vi "NXTCam-DM.vi"(0 "Input of NXTCam":T2={"Tracking Mode"=0, "Object Number to Track"=0, "Address"=2} {"Address" format="%x"; "Object Number to Track" format="%x"; "Tracking Mode" items=["Disable Tracking", "Get First Object", "Get n th Object", "Enable Tracking", "Sort Objects  by size", "Sort Objects  by Colors", "Illumination on ", "Illumination Off", "Write Colormap", "Read Colormap", "Line tracking mode", "Object Tracking mode"]}, 2 "NXT":T3={"Hardware"="NXT", "Flattened String"=""}, 3 "Input Port":T4 items=["Port 1", "Port 2", "Port 3", "Port 4"]) -> (1 "Output of NXTCam":T1, 4 "NXT dup":T3={"Hardware"="NXT", "Flattened String"=""} caption="NXT")   [LabVIEW 2011]
uses:
  <vilib>/NXT/Subs/LVHSConnector.ctl
  <vilib>/NXT/Block Support/NXT_InputPort.ctl
  <vilib>/NXT/Block Support/HWPage.SensorType.ctl
  <vilib>/NXT/Block Support/HWPage.SensorMode.ctl
panel:
  in  "Colormap Array":string="\u0000\u0000\u0000\u0000\u0000\u0000\u0000\u0000\u0000\u0000\u0000\u0000€€€€\u0000\u0000\u0000\u0000\u0000\u0000\u0000\u0000\u0000\u0000\u0000\u0000€€€€\u0000\u0000\u0000\u0000\u0000\u0000\u0000\u0000\u0000\u0000\u0000\u0000€€€€"
  in  "camera setting array":string="\u0000\u0000\u0000\u0000\u0000\u0000\u0000\u0000\u0000\u0000\u0000\u0000€€€€\u0000\u0000\u0000\u0000\u0000\u0000\u0000\u0000\u0000\u0000\u0000\u0000€€€€\u0000\u0000\u0000\u0000\u0000\u0000\u0000\u0000\u0000\u0000\u0000\u0000€€€€"
  out "Status (boolean)":bool
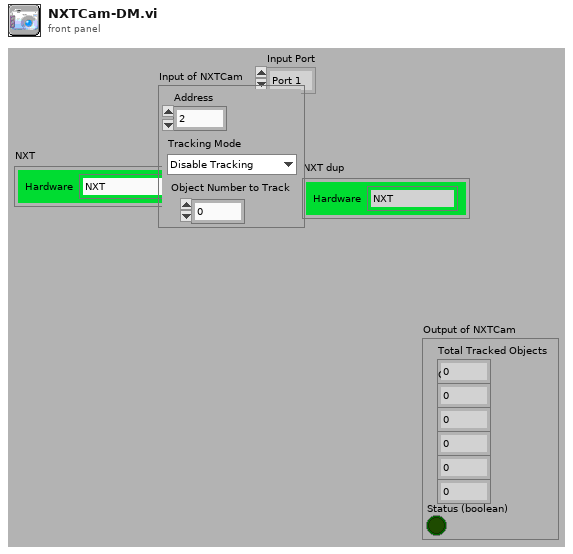
[diagram p1: front panel]
types:
  T1 = cluster{"Total Tracked Objects":u8, "Color":u8, "X Upper Left":u8, "Y Upper Left":u8, "X Lower Right":u8, "Y Lower Right":u8, "Status (boolean)":bool}
  T2 = cluster{"Tracking Mode":u8, "Object Number to Track":u8, "Address":u8}
  T3 = typedef "LVHSConnector.ctl" = cluster{"Hardware":string, "Flattened String":string}
  T4 = typedef "NXT_InputPort.ctl" = u8
  T5 = typedef "HWPage.SensorType.ctl" = u8
  T6 = typedef "HWPage.SensorMode.ctl" = u8
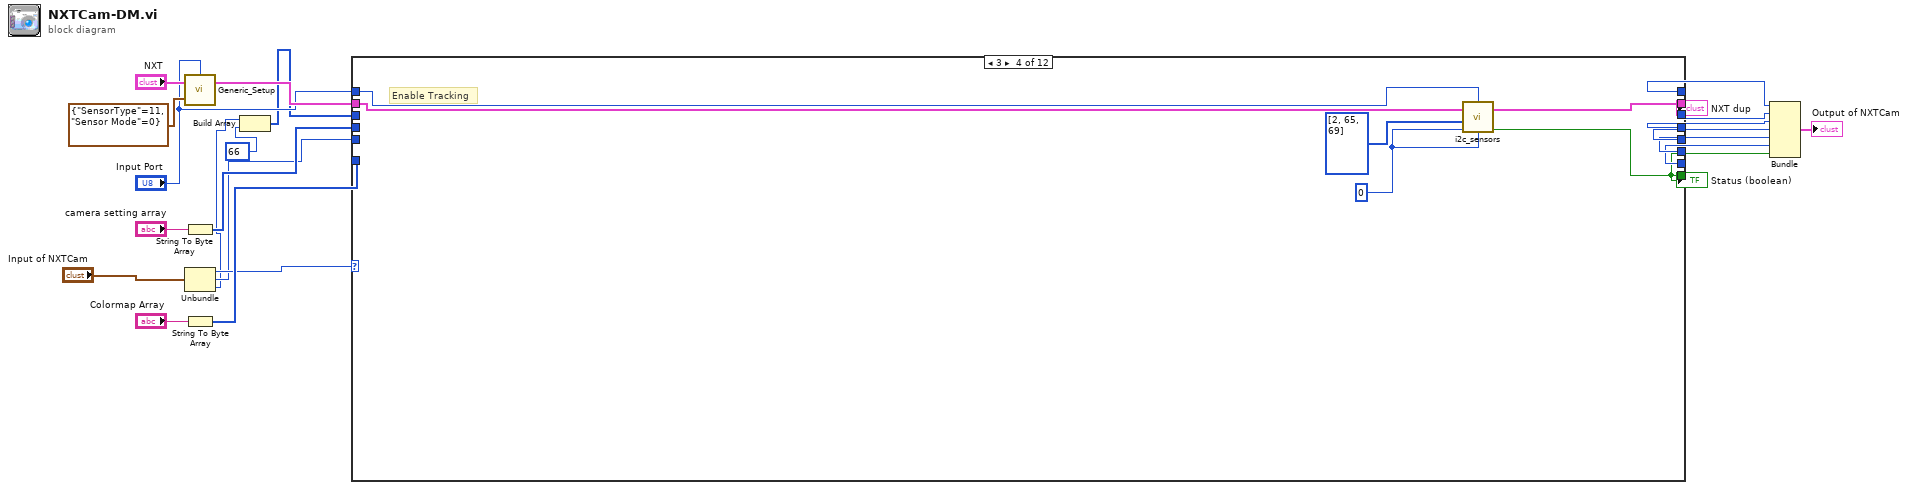
[diagram p0: block diagram]
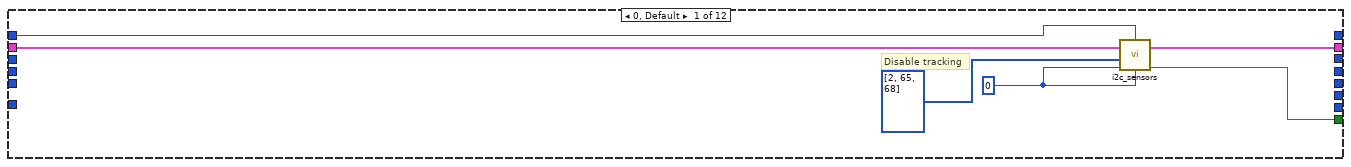
[diagram p2: hidden frame]
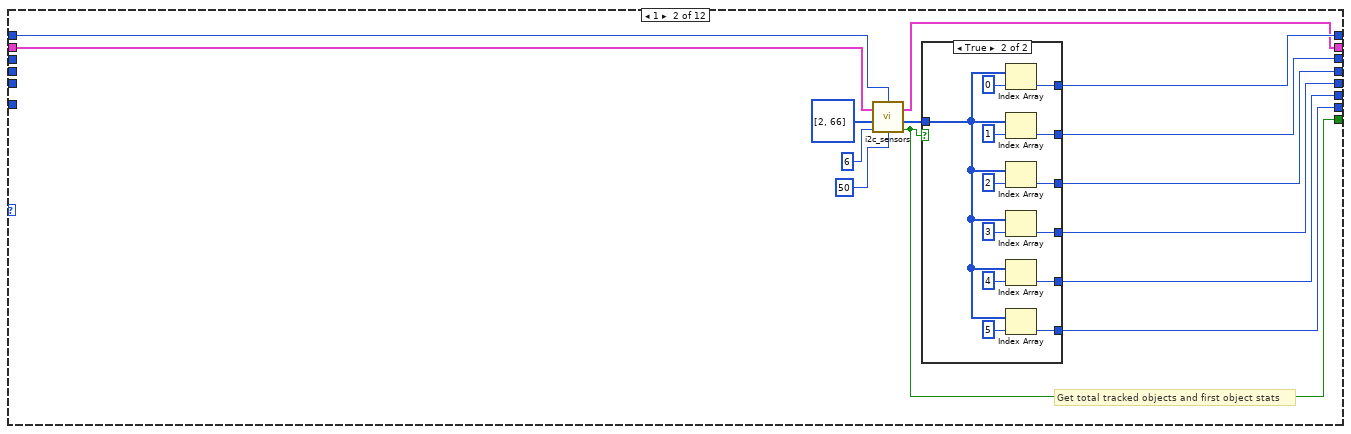
[diagram p3: hidden frame]
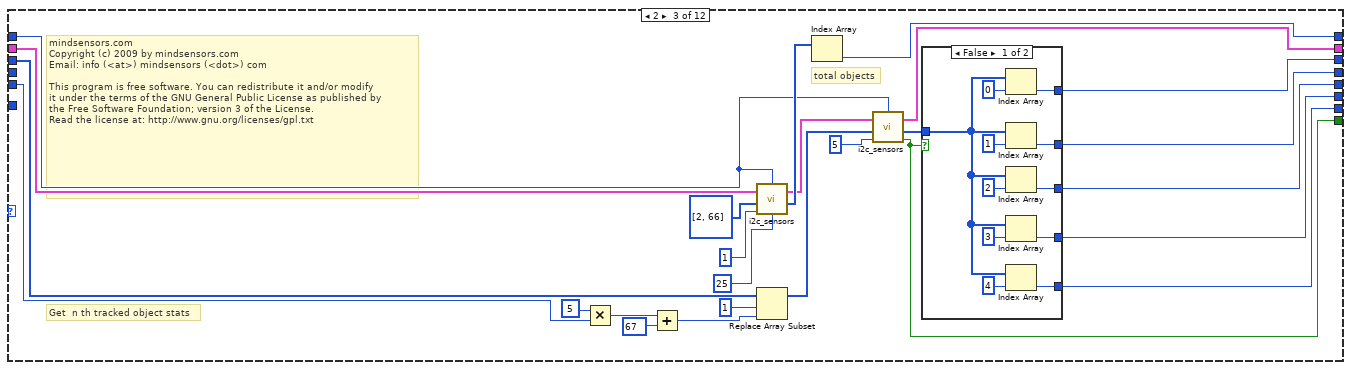
[diagram p5: hidden frame]
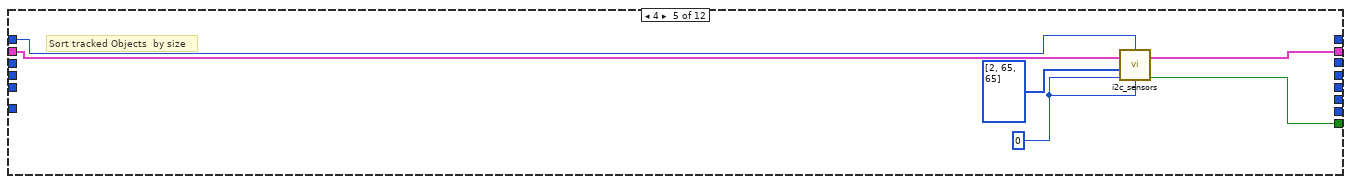
[diagram p7: hidden frame]
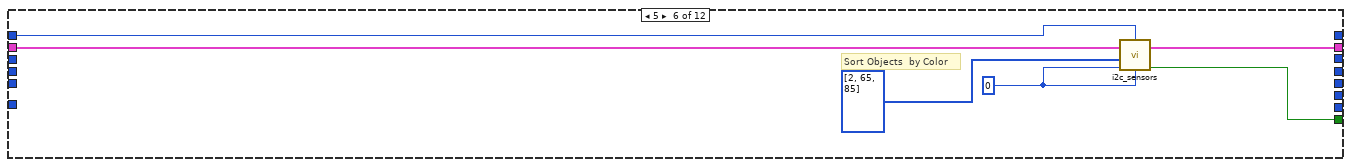
[diagram p8: hidden frame]
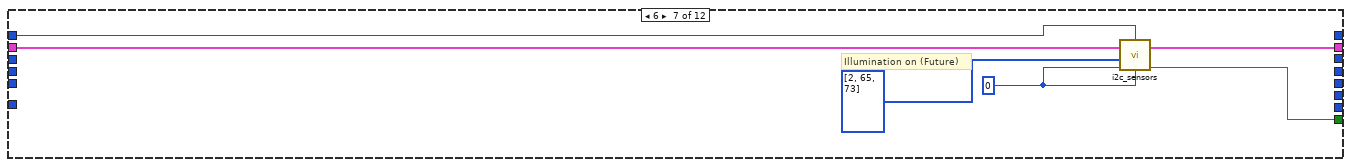
[diagram p9: hidden frame]
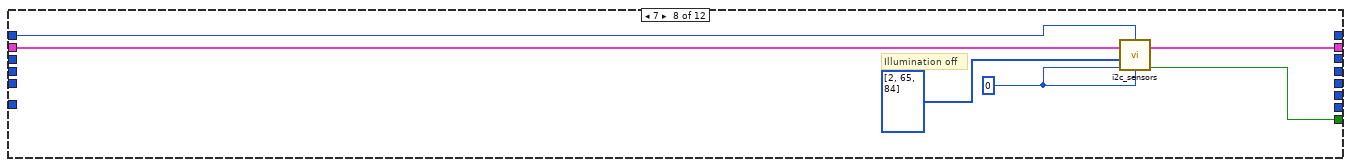
[diagram p10: hidden frame]
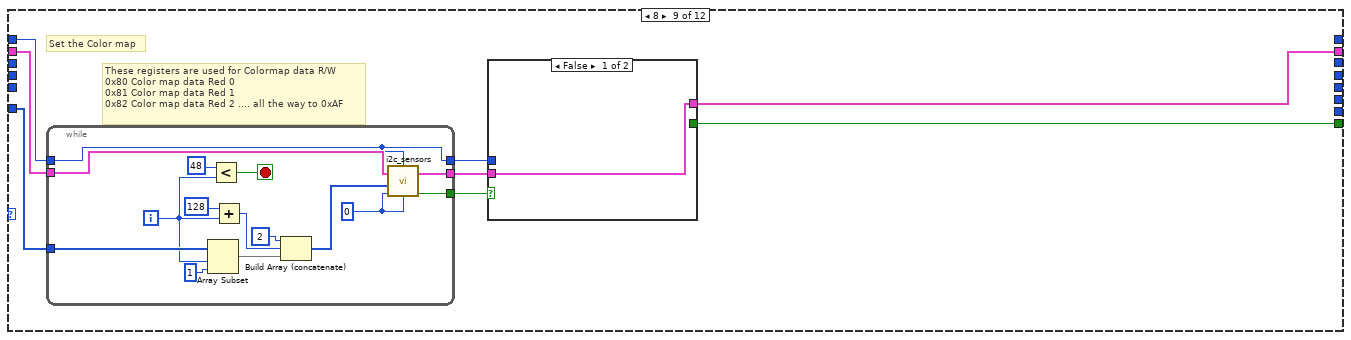
[diagram p11: hidden frame]
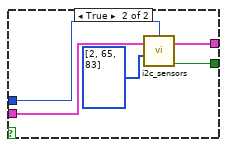
[diagram p12: hidden frame]
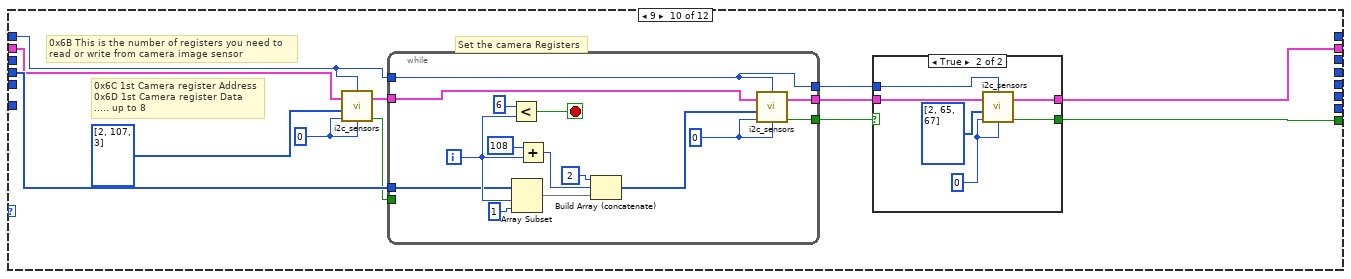
[diagram p13: hidden frame]
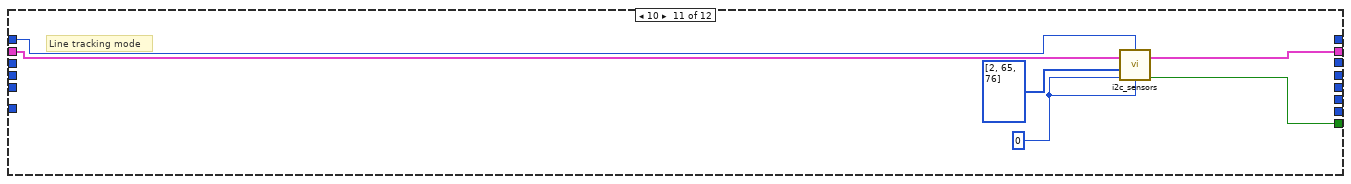
[diagram p15: hidden frame]
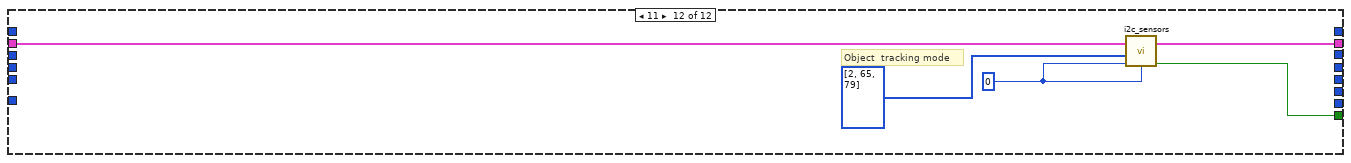
[diagram p16: hidden frame]
diagram:
  n1 = call <vilib>:"Generic_Setup.vi"("Sensor Setup"=cluster{"SensorType":T5, "Sensor Mode":T6} {"SensorType"=11, "Sensor Mode"=0}, "NXT"="NXT", "Port"="Input Port") -> ("NXT"=w15:T3)  [unwired: 1 out]
  n2 = String To Byte Array(string="camera setting array") -> (unsigned byte array=w17:u8[])
  n3 = Unbundle("Input of NXTCam") -> ("Tracking Mode"=w9:u8, "Object Number to Track"=w6:u8, "Address"=w3:u8)
  n4 = String To Byte Array(string="Colormap Array") -> (unsigned byte array=w16:u8[])
  n5 = Build Array(w3, 66 ("Slope")) -> (w1:i32[])
  n6 = case shown="3" w9 {
    tunnel: [w26 w31 w60 w94 w100 w106 w112 w118 w129 w161 w191 w193] -> w5
    tunnel: [_ w43 w70 _ _ _ _ _ _ _ _ _] -> w21
    tunnel: [_ w42 w75 _ _ _ _ _ _ _ _ _] -> w20
    tunnel: [_ w41 w74 _ _ _ _ _ _ _ _ _] -> w19
    tunnel: [_ w40 w73 _ _ _ _ _ _ _ _ _] -> w18
    tunnel: [_ w39 w72 _ _ _ _ _ _ _ _ _] -> w14
    tunnel: [_ w38 w71 _ _ _ _ _ _ _ _ _] -> w13
    tunnel: w1 -> [_ _ w76 _ _ _ _ _ _ _ _ _]
    tunnel: w16 -> [_ _ _ _ _ _ _ _ w130 _ _ _]
    tunnel: w17 -> [_ _ _ _ _ _ _ _ _ w163 _ _]
    tunnel: "Input Port" -> [w27 w33 w59 w97 w102 w107 w113 w120 w127 w157 w189 _]
    tunnel: w15 -> [w29 w36 w69 w98 w103 w110 w114 w122 w126 w159 w192 w196]
    tunnel: [w24 w35 w62 w95 w101 w109 w115 w121 w124 w152 w190 w197] -> w12
    tunnel: w6 -> [_ _ w57 _ _ _ _ _ _ _ _ _]
    frame 0, Default {
      w25 = u8 0 ("Return Length")
      # "Disable tracking"
      n7 = call <vilib>:"i2c_sensors.vi"("Return Length"=w25, "Bytes to Write"=i32[] [2, 65, 68] ("Commands"), "Wait (msec)"=w25, "NXT"=w29, "Port"=w27) -> ("Success?"=w26:bool, "NXT"=w24:T3)  [unwired: 1 out]
    }
    frame 1 {
      # "Get total tracked objects and first object stats"
      n8 = call <vilib>:"i2c_sensors.vi"("Return Length"=6 ("LS Response Length (0)"), "Bytes to Write"=i32[] [2, 66] ("Commands"), "Wait (msec)"=u32 50, "NXT"=w36, "Port"=w33) -> ("Success?"=w31:bool, "Bytes read"=w32:u8[], "NXT"=w35:T3)
      n9 = case shown="True" w31 {
        tunnel: w32 -> [_ w54]
        tunnel: [_ w55] -> w43
        tunnel: [_ w48] -> w42
        tunnel: [_ w47] -> w41
        tunnel: [_ w46] -> w40
        tunnel: [_ w45] -> w39
        tunnel: [_ w44] -> w38
        frame False {
        }
        frame True {
          n10 = Index Array(array=w54, index=0) -> (element=w55:u8)
          n11 = Index Array(array=w54, index=1) -> (element=w48:u8)
          n12 = Index Array(array=w54, index=2) -> (element=w47:u8)
          n13 = Index Array(array=w54, index=3) -> (element=w46:u8)
          n14 = Index Array(array=w54, index=4) -> (element=w45:u8)
          n15 = Index Array(array=w54, index=5) -> (element=w44:u8)
        }
      }
    }
    frame 2 {
      # "mindsensors.com\nCopyright (c) 2009 by mindsensors.com\nEmail: info (<at>) mindsensors (<dot>) com\n\nThis program is free software. You can redistribute it and/or modify\nit under the terms of the GNU General Public License as published by\nthe Free Software Foundation; version 3 of the License.\nRead the license at: http://www.gnu.org/licenses/gpl.txt"
      # "total objects"
      # "Get  n th tracked object stats"
      n16 = Multiply(x=u8 5, y=w57) -> (x*y=w81:u8)
      n17 = Add(x=w81, y=u8 67) -> (x+y=w77:u8)
      n18 = call <vilib>:"i2c_sensors.vi"("Return Length"=1 ("LS Response Length (0)"), "Bytes to Write"=i32[] [2, 66] ("Commands"), "Wait (msec)"=u32 25, "NXT"=w69, "Port"=w59) -> ("Bytes read"=w66:u8[], "NXT"=w63:T3)  [unwired: 1 out]
      n19 = Replace Array Subset(array=w76, new element=w77, index=1) -> (w64:i32[])
      n20 = Index Array(array=w66) -> (element=w70:u8)  [unwired: 1 in]
      n21 = call <vilib>:"i2c_sensors.vi"("Return Length"=5 ("LS Response Length (0)"), "Bytes to Write"=w64, "NXT"=w63, "Port"=w59) -> ("Success?"=w60:bool, "Bytes read"=w61:u8[], "NXT"=w62:T3)  [unwired: 1 in]
      n22 = case shown="False" w60 {
        tunnel: [w87 _] -> w75
        tunnel: [w86 _] -> w74
        tunnel: [w85 _] -> w73
        tunnel: [w84 _] -> w72
        tunnel: [w83 _] -> w71
        tunnel: w61 -> [w82 _]
        frame False {
          n23 = Index Array(array=w82, index=0) -> (element=w87:u8)
          n24 = Index Array(array=w82, index=1) -> (element=w86:u8)
          n25 = Index Array(array=w82, index=2) -> (element=w85:u8)
          n26 = Index Array(array=w82, index=3) -> (element=w84:u8)
          n27 = Index Array(array=w82, index=4) -> (element=w83:u8)
        }
        frame True {
        }
      }
    }
    frame 3 {
      w93 = u8 0 ("Return Length")
      # "Enable Tracking"
      n28 = call <vilib>:"i2c_sensors.vi"("Return Length"=w93, "Bytes to Write"=i32[] [2, 65, 69] ("Commands"), "Wait (msec)"=w93, "NXT"=w98, "Port"=w97) -> ("Success?"=w94:bool, "NXT"=w95:T3)  [unwired: 1 out]
    }
    frame 4 {
      w99 = u8 0 ("Return Length")
      # "Sort tracked Objects  by size"
      n29 = call <vilib>:"i2c_sensors.vi"("Return Length"=w99, "Bytes to Write"=i32[] [2, 65, 65] ("Commands"), "Wait (msec)"=w99, "NXT"=w103, "Port"=w102) -> ("Success?"=w100:bool, "NXT"=w101:T3)  [unwired: 1 out]
    }
    frame 5 {
      w105 = u8 0 ("Return Length")
      # "Sort Objects  by Color"
      n30 = call <vilib>:"i2c_sensors.vi"("Return Length"=w105, "Bytes to Write"=i32[] [2, 65, 85] ("Commands"), "Wait (msec)"=w105, "NXT"=w110, "Port"=w107) -> ("Success?"=w106:bool, "NXT"=w109:T3)  [unwired: 1 out]
    }
    frame 6 {
      w111 = u8 0 ("Return Length")
      # "Illumination on (Future)"
      n31 = call <vilib>:"i2c_sensors.vi"("Return Length"=w111, "Bytes to Write"=i32[] [2, 65, 73] ("Commands"), "Wait (msec)"=w111, "NXT"=w114, "Port"=w113) -> ("Success?"=w112:bool, "NXT"=w115:T3)  [unwired: 1 out]
    }
    frame 7 {
      w117 = u8 0 ("Return Length")
      # "Illumination off"
      n32 = call <vilib>:"i2c_sensors.vi"("Return Length"=w117, "Bytes to Write"=i32[] [2, 65, 84] ("Commands"), "Wait (msec)"=w117, "NXT"=w122, "Port"=w120) -> ("Success?"=w118:bool, "NXT"=w121:T3)  [unwired: 1 out]
    }
    frame 8 {
      # "These registers are used for Colormap data R/W\n0x80 Color map data Red 0 \n0x81 Color map data Red 1 \n0x82 Color map data Red 2 .... all the way to 0xAF"
      # "Set the Color map"
      n33 = while {
        tunnel: w130 -> [w151]
        tunnel: w127 -> [w141]
        tunnel: [w141] -> w128
        tunnel: w126 -> [w142]
        tunnel: [w139] -> w125
        tunnel: [w137] -> w123
        i -> [w146]
        stop <- w147 stop-if-true
        w138 = u8 0 ("Return Length")
        n34 = Array Subset(array=w151, index=w146, length=1) -> (w143:u8[])
        n35 = Less?(x=48, y=w146) -> (x < y?=w147:bool)
        n36 = Add(x=u8 128 ("register"), y=w146) -> (x+y=w144:i32)
        n37 = Build Array (concatenate)(2 ("Slope"), w144, w143) -> (w140:i32[])
        n38 = call <vilib>:"i2c_sensors.vi"("Return Length"=w138, "Bytes to Write"=w140, "Wait (msec)"=w138, "NXT"=w142, "Port"=w141) -> ("Success?"=w137:bool, "NXT"=w139:T3)  [unwired: 1 out]
      }
      n39 = case shown="False" w123 {
        tunnel: [_ w135] -> w129
        tunnel: w128 -> [_ w136]
        tunnel: w125 -> [w131 w134]
        tunnel: [w131 w132] -> w124
        frame False {
        }
        frame True {
          n40 = call <vilib>:"i2c_sensors.vi"("Bytes to Write"=i32[] [2, 65, 83] ("Commands"), "NXT"=w134, "Port"=w136) -> ("Success?"=w135:bool, "NXT"=w132:T3)  [unwired: 2 in, 1 out]
        }
      }
    }
    frame 9 {
      w153 = u8 0 ("Return Length")
      # "0x6C 1st Camera register Address\n0x6D 1st Camera register Data\n..... up to 8"
      # "0x6B This is the number of registers you need to\nread or write from camera image sensor"
      # "Set the camera Registers"
      n41 = call <vilib>:"i2c_sensors.vi"("Return Length"=w153, "Bytes to Write"=i32[] [2, 107, 3] ("Commands"), "Wait (msec)"=w153, "NXT"=w159, "Port"=w157) -> ("Success?"=w156:bool, "NXT"=w155:T3)  [unwired: 1 out]
      n42 = while {
        tunnel: w163 -> [w181]
        tunnel: [w174] -> w162
        tunnel: w156 -> [_]
        tunnel: w157 -> [w173]
        tunnel: [w173] -> w160
        tunnel: w155 -> [w176]
        tunnel: [w175] -> w154
        i -> [w182]
        stop <- w183 stop-if-true
        w172 = u8 0 ("Return Length")
        n43 = Less?(x=6, y=w182) -> (x < y?=w183:bool)
        n44 = Array Subset(array=w181, index=w182, length=1) -> (w178:u8[])
        n45 = Add(x=u8 108 ("register"), y=w182) -> (x+y=w179:i32)
        n46 = Build Array (concatenate)(2 ("Slope"), w179, w178) -> (w177:i32[])
        n47 = call <vilib>:"i2c_sensors.vi"("Return Length"=w172, "Bytes to Write"=w177, "Wait (msec)"=w172, "NXT"=w176, "Port"=w173) -> ("Success?"=w174:bool, "NXT"=w175:T3)  [unwired: 1 out]
      }
      n48 = case shown="True" w162 {
        selector: w162 -> [w165 _]
        tunnel: [w165 w169] -> w161
        tunnel: w160 -> [_ w166]
        tunnel: w154 -> [w164 w168]
        tunnel: [w164 w167] -> w152
        frame False {
        }
        frame True {
          w170 = u8 0 ("Return Length")
          n49 = call <vilib>:"i2c_sensors.vi"("Return Length"=w170, "Bytes to Write"=i32[] [2, 65, 67] ("Commands"), "Wait (msec)"=w170, "NXT"=w168, "Port"=w166) -> ("Success?"=w169:bool, "NXT"=w167:T3)  [unwired: 1 out]
        }
      }
    }
    frame 10 {
      w188 = u8 0 ("Return Length")
      # "Line tracking mode"
      n50 = call <vilib>:"i2c_sensors.vi"("Return Length"=w188, "Bytes to Write"=i32[] [2, 65, 76] ("Commands"), "Wait (msec)"=w188, "NXT"=w192, "Port"=w189) -> ("Success?"=w191:bool, "NXT"=w190:T3)  [unwired: 1 out]
    }
    frame 11 {
      w194 = u8 0 ("Return Length")
      # "Object  tracking mode"
      n51 = call <vilib>:"i2c_sensors.vi"("Return Length"=w194, "Bytes to Write"=i32[] [2, 65, 79] ("Commands"), "Wait (msec)"=w194, "NXT"=w196) -> ("Success?"=w193:bool, "NXT"=w197:T3)  [unwired: 1 in, 1 out]
    }
  }
  "NXT dup" <- w12
  "Status (boolean)" <- w5
  n52 = Bundle(w21, w20, w19, w18, w14, w13, "Success?"=w5) -> (→"Output of NXTCam":cluster{u8, u8, u8, u8, u8, u8, "Success?":bool})  [unwired: 1 out]
